vi "pl1000Run.vi"(6 "method":enum16{"BM_SINGLE", "BM_WINDOW", "BM_STREAM"}(ring), 8 "error in (no error)":errorcluster, 10 "noOfValues":u32, 11 "pl1000 handle":i16) -> (0 "error out":errorcluster, 3 "pl1000 handle out":i16)   [LabVIEW 2010]
doc: "This function tells the unit to start capturing data\n\nno_of_values: the total number of samples to be collected across all channels\n\nmethod: which method to use to collect the data, from the following list:\nBM_SINGLE\nBM_WINDOW\nBM_STREAM"
uses:
  pl1000.dll
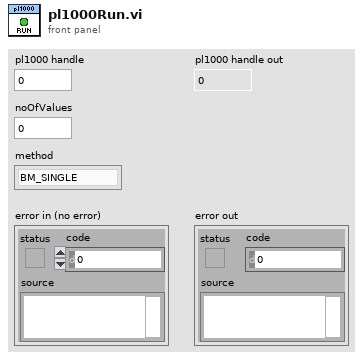
[diagram p1: front panel]
types:
  T1 = cluster{"status":bool, "code":u32, "source":string}
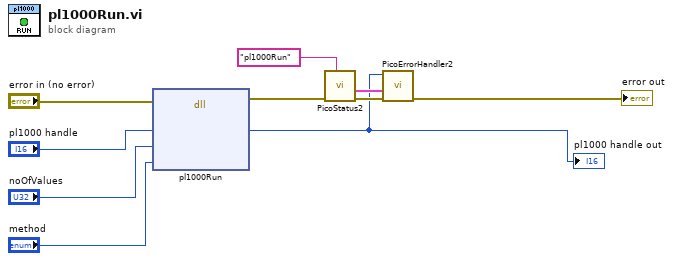
[diagram p0: block diagram]
diagram:
  n1 = dll-call lib="pl1000.dll" fn="pl1000Run"(error in="error in (no error)", "handle"="pl1000 handle", "noOfValues"="noOfValues", "method"="method") -> (error out=w3:errorcluster, "handle"=w2:i16)  [unwired: 5 in, 1 out]
  "pl1000 handle out" <- w2
  n2 = call "PicoStatus2.vi"("PICO source"="pl1000Run", "Error in"=w3) -> ("error out"=w6:errorcluster, "PICO_STATUS out"=w5:T1)  [unwired: 6 in]
  n3 = call "PicoErrorHandler2.vi"("error in (no error)"=w6, "PICO_STATUS in"=w5, "handle In"=w2) -> ("error out"=→"error out":errorcluster)  [unwired: 8 in]
